vi "Read Config Ref.vi"(8 "error in (no error)":errorcluster, 11 "Base In":refnum<class "Base.lvclass">) -> (0 "error out":errorcluster, 2 "Config File Refnum":variant, 3 "Base Out":refnum<class "Base.lvclass">)   [LabVIEW 2020, in "Base.lvclass"]
doc: "For the configuration interface to work, the class implementing the interface needs to save the reference to the file in the class attributes. This is an accessor for that attribute which must be implemented by the class."
uses:
  Base.lvclass
  Base.lvclass/Base.ctl
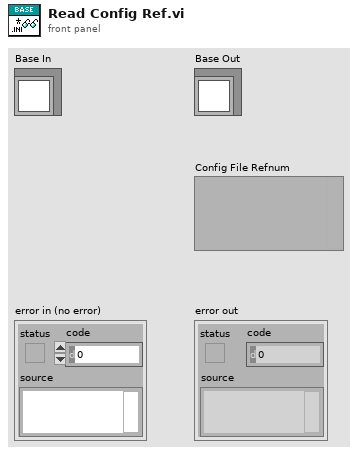
[diagram p1: front panel]
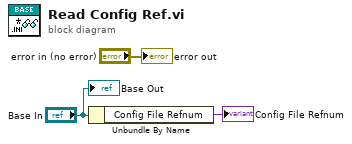
[diagram p0: block diagram]
diagram:
  n1 = Unbundle By Name("Base In") -> ("Config File Refnum"=→"Config File Refnum":variant)
  "error out" <- "error in (no error)"
  "Base Out" <- "Base In"
